vi "test_KVP to Variant.vi"(8 "error in (no error)":errorcluster) -> (0 "error out":errorcluster)   [LabVIEW 2013]
uses:
  <vilib>/addons/_JKI Toolkits/Caraya/classes/Assert/Assert Equal Value and Type_Variant.vi
  <vilib>/addons/_JKI Toolkits/Caraya/classes/Test/Test.lvclass
  <vilib>/addons/_JKI Toolkits/Caraya/classes/Assert/Assert.lvclass
  source/Variant/OpenVariant.lvlib
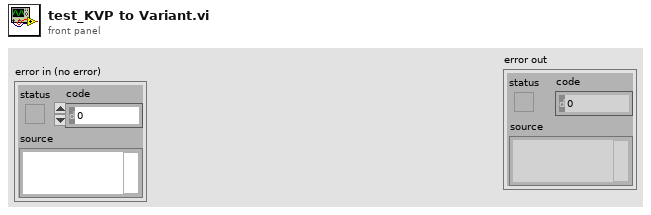
[diagram p1: front panel]
types:
  T1 = cluster{"status":bool, "source":string, "error":cluster{"status":bool, "code":i32, "source":string, "new value":i32}, "code":i32}
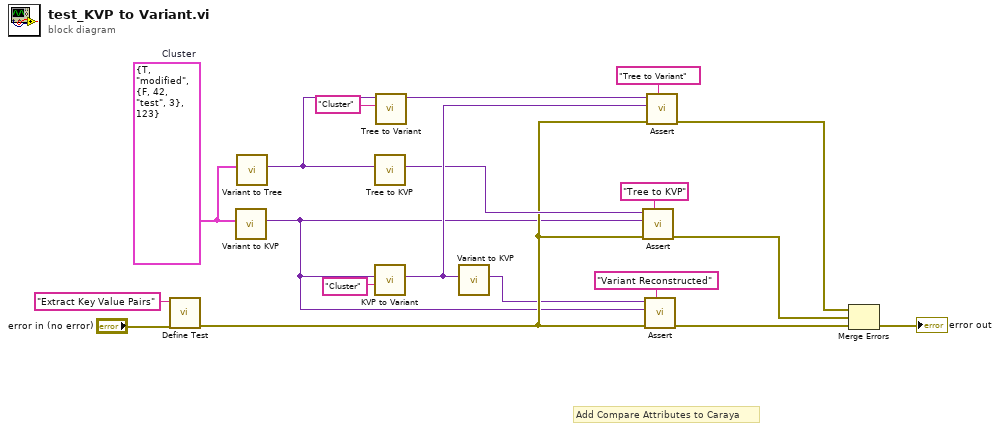
[diagram p0: block diagram]
diagram:
  w14 = T1 {"status"=TRUE, "source"="modified", "error"={"status"=FALSE, "code"=42, "source"="test", "new value"=3}, "code"=123}  # Cluster
  # "Add Compare Attributes to Caraya"
  n1 = call <vilib>:"Define Test.vi"("error in (no error)"="error in (no error)", "Label (VI Title)"="Extract Key Value Pairs") -> ("error out"=w4:errorcluster)  [unwired: 9 in]
  n2 = call "Variant to KVP.vi"("Variant"=w14) -> ("KVP Dictionary"=w2:variant)  [unwired: 10 in]
  n3 = call "Variant to Tree.vi"("Variant"=w14) -> ("Variant Tree"=w9:variant)  [unwired: 10 in]
  n4 = call "Tree to KVP.vi"("Variant Tree"=w9) -> ("KVP"=w10:variant)  [unwired: 10 in]
  n5 = call "KVP to Variant.vi"("Name"="Cluster" ("Label (VI Title)"), "KVP"=w2) -> ("Reconstructed Data"=w11:variant)  [unwired: 9 in]
  n6 = call "Tree to Variant.vi"("Name"="Cluster" ("Label (VI Title)"), "Variant Tree"=w9) -> ("Variant"=w7:variant)  [unwired: 9 in]
  n7 = call "Variant to KVP.vi"("Variant"=w11) -> ("KVP Dictionary"=w1:variant)  [unwired: 10 in]
  n8 = call-poly <vilib>:"Assert.vi"("Label"="Tree to KVP" ("Label (VI Title)"), "error in (no error)"=w4, "Y"=w2, "X"=w10) -> ("error out"=w6:errorcluster)  [unwired: 7 in]
  n9 = call-poly <vilib>:"Assert.vi"("Label"="Variant Reconstructed" ("Label (VI Title)"), "error in (no error)"=w4, "Y"=w2, "X"=w1) -> ("error out"=w5:errorcluster)  [unwired: 7 in]
  n10 = call-poly <vilib>:"Assert.vi"("Label"="Tree to Variant" ("Label (VI Title)"), "error in (no error)"=w4, "Y"=w11, "X"=w7) -> ("error out"=w3:errorcluster)  [unwired: 7 in]
  n11 = Merge Errors(w3, w6, w5) -> (→"error out":errorcluster)
